vi "_io_read_errors.vi"(8 "error in":errorcluster caption="error in (no error)", 10 "Custom Timeout (VISA Timeout)":i32=-1, 11 "VISA resource name":refnum<visa-resource-name>) -> (0 "error out":errorcluster, 3 "VISA resource name out":refnum<visa-resource-name>)   [LabVIEW 2022 SP3, in "hmp4000_rsidr_core.lvlib"]
uses:
  hmp4000_rsidr_core.lvlib
  type_Error_Codes.ctl
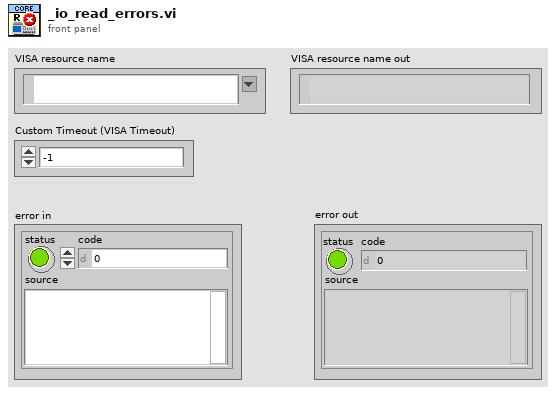
[diagram p1: front panel]
types:
  T1 = typedef "hmp4000_rsidr_core.lvlib/type_Error_Codes.ctl" = enum16{"No_error", "VISA_err_ResourceNotFound", "VISA_err_Timeout", "VISA_warn_MoreDataAvailable", "RS_err_MissingCallback", "RS_err_InvalidAttribute", "RS_err_InvalidValue", "RS_err_UnknownResource", "RS_err_AlreadyInitialized", "RS_err_InstrumentStatus", "RS_err_BadRepCapName", "RS_err_TypesMismatch", "RS_err_ValueNotSupported", "RS_err_InvalidRngTable", "RS_err_IDqueryFail", "RS_err_UnexpResponse", "VISA_warn_ConfigNotLoaded", "RS_err_AttributeNotReadable", "RS_err_AttributeNotWritable", "RS_err_InstrumentType", "RS_err_InstrumentOption", "VISA_err_InvalidSize", "RS_err_ReliabilityIndicator", "VISA_warn_UnknownStatus", "VISA_warn_TermCharRead", "VISA_err_IO_error", "RS_err_FunctionNotSupported", "VISA_warn_QueueEmpty"}
  T2 = typedef "hmp4000_rsidr_core.lvlib/type_Session_Data.ctl" = cluster{"IDN string":string, "Instrument FW":string, "Instr type":string, "Instr type for err. msg.":string, "Installed Options":string[], "Ignore Error Messages":string, "Logging params":variant, "OPC Timeout":i32, "VISA Timeout":i32, "STB Poll VISA Timeout":i32, "Additional Flags":i32, "Wait Before Read":i32, "Wait Before Write":i32, "Option String Flags":i32, "IO Segment Size":i64, "VISA Access Mode":T3, "Interface Type":T4, "OPC Wait Mode":T5, "Bin Float Number  Format":T6, "Bin Integer Number Format":T7, "Simulate":bool, "VXIcapable":bool, "Duplicate Session":bool, "Add LF to Write":bool, "Logging":bool, "Fast Sweep":bool, "Query Instrument Status":bool, "Check Range":bool, "Check Options":bool}
  T3 = typedef "hmp4000_rsidr_core.lvlib/type_VisaAccessMode.ctl" = u16
  T4 = typedef "hmp4000_rsidr_core.lvlib/type_InterfaceType.ctl" = enum16{"Unknown", "GPIB", "VXI", "GPIB_VXI", "ASRL", "PXI", "TCPIP", "USB", "SOCKET"}
  T5 = typedef "hmp4000_rsidr_core.lvlib/type_OPC_Wait_Mode.ctl" = enum16{"STBpolling", "STBpollingSlow", "STBpollingSuperSlow", "ServiceRequest", "OPCquery"}
  T6 = typedef "hmp4000_rsidr_core.lvlib/type_Binary_Float_Number_Format.ctl" = enum16{"Float_4_Bytes_Swapped", "Float_4_Bytes", "Double_8_Bytes_Swapped", "Double_8_Bytes"}
  T7 = typedef "hmp4000_rsidr_core.lvlib/type_Binary_Integer_Number_Format.ctl" = enum16{"Int32_4_Bytes_Swapped", "Int32_4 Bytes", "Int16_2_Bytes_Swapped", "Int16_2_Bytes"}
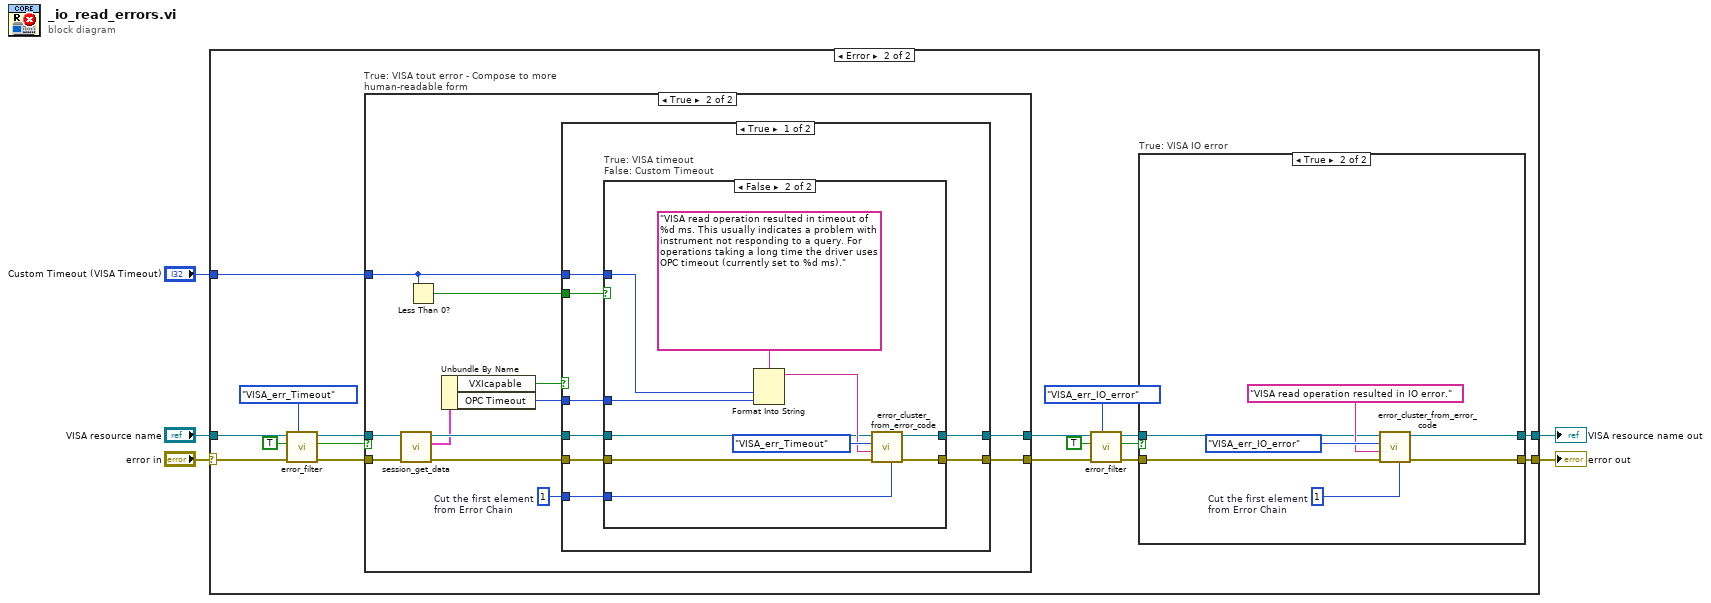
[diagram p0: block diagram]
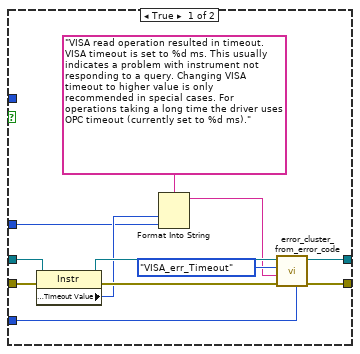
[diagram p5: hidden frame]
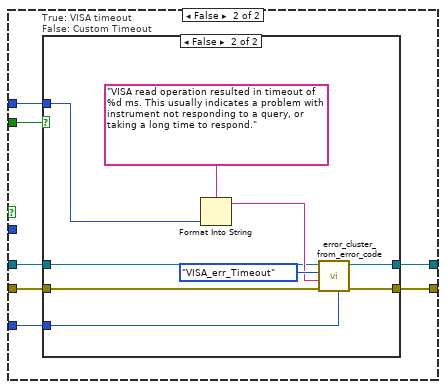
[diagram p6: hidden frame]
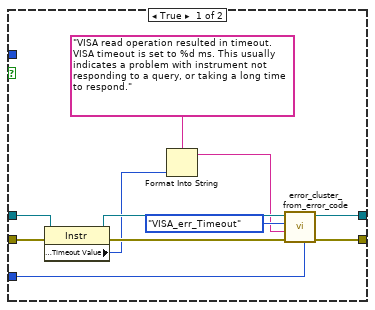
[diagram p7: hidden frame]
diagram:
  n1 = case shown="Error" "error in" {
    selector: "error in" -> [w7 w20]
    tunnel: [w7 w9] -> w3
    tunnel: "VISA resource name" -> [w6 w19]
    tunnel: [w6 w10] -> w2
    tunnel: "Custom Timeout (VISA Timeout)" -> [_ w8]
    frame No Error {
    }
    frame Error {
      n2 = call "error_filter.vi"("Error Enum in"=type_Error_Codes."VISA_err_Timeout" ("Code to detect"), "error in"=w20, "Clear detected code (F)"=TRUE, "VISA resource name"=w19) -> ("error out"=w22:errorcluster, "Code Detected"=w21:bool, "VISA resource name out"=w18:refnum<visa-resource-name>)  [unwired: 5 in]
      n3 = case "True: VISA tout error - Compose to more human-readable form" shown="True" w21 {
        tunnel: w22 -> [w35 w45]
        tunnel: [w35 w47] -> w15
        tunnel: [w34 w46] -> w16
        tunnel: w18 -> [w34 w42]
        tunnel: w8 -> [_ w37]
        frame False {
        }
        frame True {
          w38 = 1  # Cut the first element from Error Chain
          n4 = call "session_get_data.vi"("error in"=w45, "VISA resource name"=w42) -> ("error out"=w44:errorcluster, "Session User Data out"=w41:T2, "VISA resource name out"=w43:refnum<visa-resource-name>)  [unwired: 6 in, 1 out]
          n5 = Less Than 0?(x=w37) -> (x < 0?=w36:bool)
          n6 = Unbundle By Name(w41) -> ("VXIcapable"=w39:bool, "OPC Timeout"=w40:i32)
          n7 = case shown="True" w39 {
            tunnel: [w55 w84] -> w47
            tunnel: [w54 w83] -> w46
            tunnel: w44 -> [w53 w82]
            tunnel: w43 -> [w52 w81]
            tunnel: w40 -> [w51 _]
            tunnel: w38 -> [w50 w80]
            tunnel: w37 -> [w48 w78]
            tunnel: w36 -> [w49 w79]
            frame True {
              n8 = case "True: VISA timeout\nFalse: Custom Timeout" shown="False" w49 {
                tunnel: [w66 w76] -> w55
                tunnel: [w65 w75] -> w54
                tunnel: w53 -> [w59 w70]
                tunnel: w52 -> [w58 w69]
                tunnel: w51 -> [w57 w72]
                tunnel: w50 -> [w56 w71]
                tunnel: w48 -> [_ w68]
                frame True {
                  n9 = property on="Property Node" class="Instr"(reference=w58, error in=w59) -> (reference out=w63:refnum<visa-resource-name>, error out=w64:errorcluster, "General Settings:Timeout Value"=w62:u32)
                  n10 = Format Into String(format string="VISA read operation resulted in timeout. VISA timeout is set to %d ms. This usually indicates a problem with instrument not responding to a query. Changing VISA timeout to higher value is only recommended in special cases. For operations taking a long time the driver uses OPC timeout (currently set to %d ms).", w62, w57) -> (resulting string=w61:string)  [unwired: 2 in, 1 out]
                  n11 = call "error_cluster_from_error_code.vi"("Cut first x elements\nfrom Error Chain (0)"=w56, "error in"=w64, "Error Message (\"\")"=w61, "Error Enum in"=type_Error_Codes."VISA_err_Timeout", "VISA resource name"=w63) -> ("error out"=w66:errorcluster, "VISA resource name out"=w65:refnum<visa-resource-name>)  [unwired: 5 in]
                }
                frame False {
                  n12 = Format Into String(format string="VISA read operation resulted in timeout of %d ms. This usually indicates a problem with instrument not responding to a query. For operations taking a long time the driver uses OPC timeout (currently set to %d ms).", w68, w72) -> (resulting string=w74:string)  [unwired: 2 in, 1 out]
                  n13 = call "error_cluster_from_error_code.vi"("Cut first x elements\nfrom Error Chain (0)"=w71, "error in"=w70, "Error Message (\"\")"=w74, "Error Enum in"=type_Error_Codes."VISA_err_Timeout", "VISA resource name"=w69) -> ("error out"=w76:errorcluster, "VISA resource name out"=w75:refnum<visa-resource-name>)  [unwired: 5 in]
                }
              }
            }
            frame False {
              n14 = case "True: VISA timeout\nFalse: Custom Timeout" shown="False" w79 {
                tunnel: [w94 w103] -> w84
                tunnel: [w93 w102] -> w83
                tunnel: w82 -> [w87 w97]
                tunnel: w81 -> [w86 w98]
                tunnel: w80 -> [w85 w99]
                tunnel: w78 -> [_ w96]
                frame True {
                  n15 = property on="Property Node" class="Instr"(reference=w86, error in=w87) -> (reference out=w91:refnum<visa-resource-name>, error out=w92:errorcluster, "General Settings:Timeout Value"=w90:u32)
                  n16 = Format Into String(format string="VISA read operation resulted in timeout. VISA timeout is set to %d ms. This usually indicates a problem with instrument not responding to a query, or taking a long time to respond.", w90) -> (resulting string=w89:string)  [unwired: 2 in, 1 out]
                  n17 = call "error_cluster_from_error_code.vi"("Cut first x elements\nfrom Error Chain (0)"=w85, "error in"=w92, "Error Message (\"\")"=w89, "Error Enum in"=type_Error_Codes."VISA_err_Timeout", "VISA resource name"=w91) -> ("error out"=w94:errorcluster, "VISA resource name out"=w93:refnum<visa-resource-name>)  [unwired: 5 in]
                }
                frame False {
                  n18 = Format Into String(format string="VISA read operation resulted in timeout of %d ms. This usually indicates a problem with instrument not responding to a query, or taking a long time to respond.", w96) -> (resulting string=w101:string)  [unwired: 2 in, 1 out]
                  n19 = call "error_cluster_from_error_code.vi"("Cut first x elements\nfrom Error Chain (0)"=w99, "error in"=w97, "Error Message (\"\")"=w101, "Error Enum in"=type_Error_Codes."VISA_err_Timeout", "VISA resource name"=w98) -> ("error out"=w103:errorcluster, "VISA resource name out"=w102:refnum<visa-resource-name>)  [unwired: 5 in]
                }
              }
            }
          }
        }
      }
      n20 = call "error_filter.vi"("Error Enum in"=type_Error_Codes."VISA_err_IO_error" ("Code to detect"), "error in"=w15, "Clear detected code (F)"=TRUE, "VISA resource name"=w16) -> ("error out"=w12:errorcluster, "Code Detected"=w11:bool, "VISA resource name out"=w13:refnum<visa-resource-name>)  [unwired: 5 in]
      n21 = case "True: VISA IO error" shown="True" w11 {
        tunnel: w12 -> [w25 w28]
        tunnel: [w26 w33] -> w10
        tunnel: w13 -> [w26 w29]
        tunnel: [w25 w32] -> w9
        frame False {
        }
        frame True {
          w27 = 1  # Cut the first element from Error Chain
          n22 = call "error_cluster_from_error_code.vi"("Cut first x elements\nfrom Error Chain (0)"=w27, "error in"=w28, "Error Message (\"\")"="VISA read operation resulted in IO error.", "Error Enum in"=type_Error_Codes."VISA_err_IO_error", "VISA resource name"=w29) -> ("error out"=w32:errorcluster, "VISA resource name out"=w33:refnum<visa-resource-name>)  [unwired: 5 in]
        }
      }
    }
  }
  "VISA resource name out" <- w2
  "error out" <- w3
